vi "myRIO_BRig_FPGA_v3,2__PortC.vi"() -> ()   [LabVIEW 2014]
uses:
  <vilib>/rvi/FXPMathLib/FxpDiv/subVIs/nifxpmath_Div_SimConfig.ctl
  <vilib>/rvi/FXPMathLib/FxpSinAndCos/subVIs/nifxpmath_SinAndCos_SimConfig.ctl
  <vilib>/rvi/FXPMathLib/FxpDiv/simVIs/DllFxpDivTemp_sub.vi
  <vilib>/rvi/FXPMathLib/FxpSinAndCos/simVIs/DllFxpSinAndCosTemp_sub.vi
  <vilib>/rvi/Emulation/niFpgaGetClockAttributes.vi
  <vilib>/rvi/Emulation/niFpgaSctlEmulationGetInTimedLoop.vi
  <vilib>/rvi/Emulation/niFpgaEmulationReportErrorSimple.vi
  <vilib>/rvi/eio/common/nirviEmuTemplateMethod_errors.vi
  <vilib>/rvi/Emulation/niFpgaCriticalErrorInLSC.vi
  <vilib>/rvi/FXPMathLib/FxpDiv/XNode/nifxpmath_Div.xnode
  <vilib>/rvi/FXPMathLib/FxpMul/XNode/nifxpmath_Multiplier.xnode
  <vilib>/rvi/FXPMathLib/FxpSinAndCos/XNode/nifxpmath_SinAndCos.xnode
  <vilib>/rvi/FXPMathLib/FxpSub/XNode/nifxpmath_Sub.xnode
  <vilib>/eio/EIONode/EIONode.xnode
  <vilib>/rvi/FXPMathLib/sim/FxpSim.dll
panel:
  in  "AO0":i16
  in  "f_time_select":u32=173
  in  "laser_Nvalley":u32=100
  in  "laser_Npeak":u32=100
  in  "laserledMTrig":bool
  in  "tCycle_laser_wro":u32=100
  in  "tDelay_laser_wro":u32
  in  "tCycle_laser_rew":u32=100
  in  "tDelay_laser_rew":u32
  in  "laserResponse_reward_LED":bool
  in  "laserResponse_wrong_LED":bool
  out "SelectWrong":bool
  out "SelectReward":bool
  in  "laserResponse_wrong":bool
  in  "laserResponse_reward":bool
  in  "Left(F)_or_Right(T)":bool
  in  "ignoreWrong":bool
  in  "SelectionState":bool
  in  "laserMTrig":bool
  in  "FPGA_Stop":bool
  in  "audioTrigger_L":bool
  in  "audioTrigger_R":bool
  in  "audioFreq_L_Hz":u16=1000 min=1000 max=14000 step=1000
  in  "audioAmp_L":u16=1 min=1 max=32767 step=1
  in  "audioFreq_R_Hz":u16=1000 min=1000 max=14000 step=1000
  in  "audioAmp_R":u16=1 min=1 max=32767 step=1
  in  "A3_SL":bool
  in  "A1_SR":bool
  in  "Counts_Reset":bool
  out "A4_LickR":u32
  out "A2_LickL":u32
  in  "A6_Act":bool
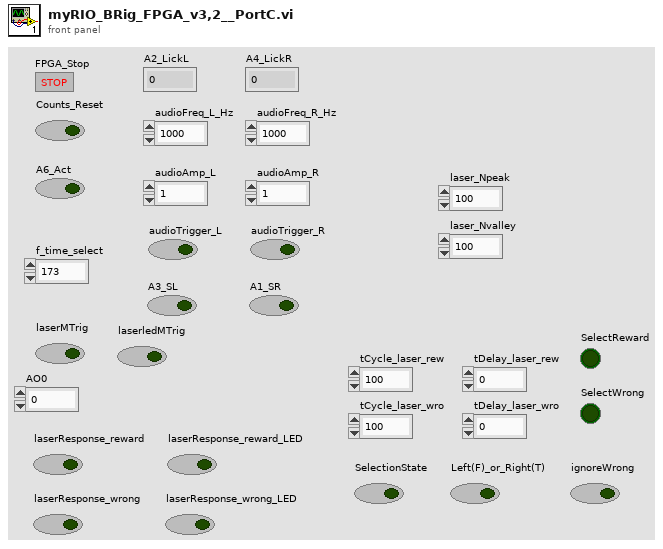
[diagram p1: front panel]
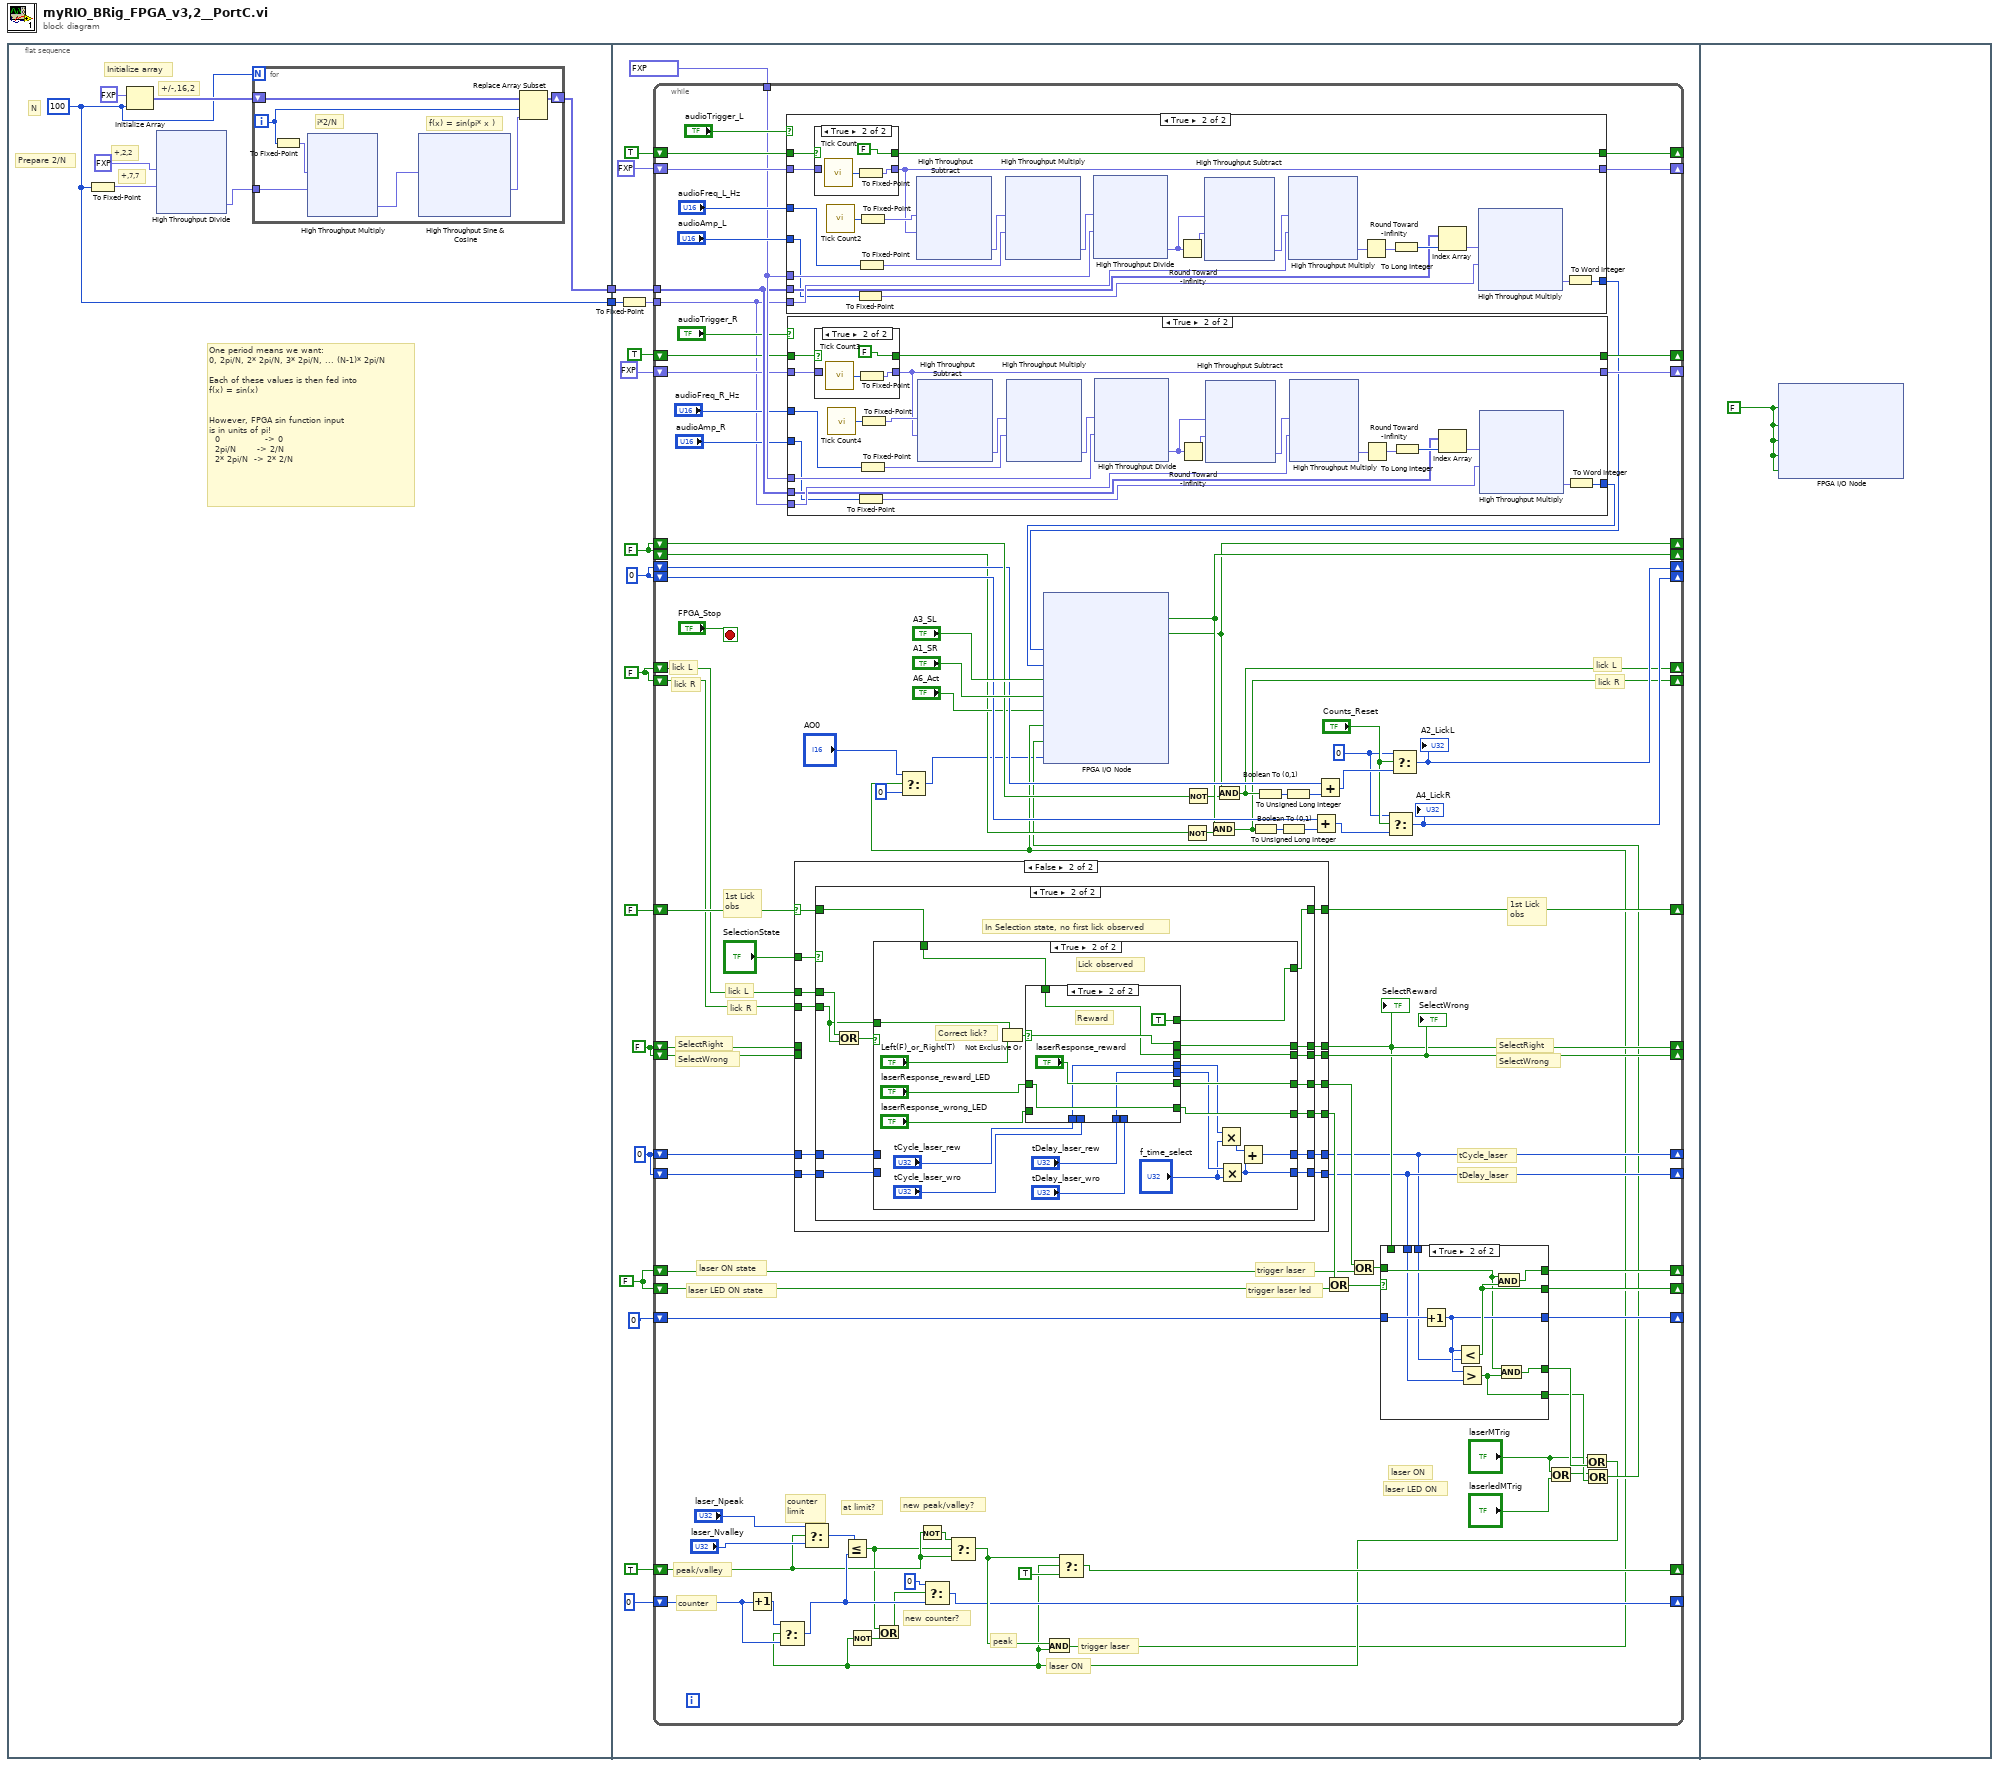
[diagram p0: block diagram]
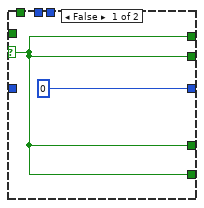
[diagram p2: hidden frame]
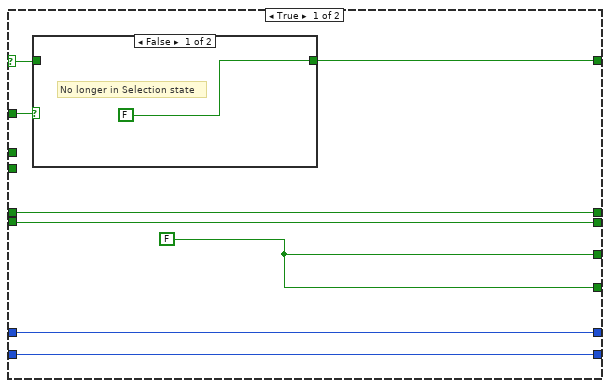
[diagram p3: hidden frame]
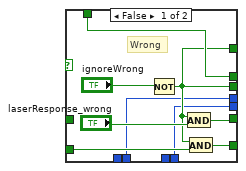
[diagram p7: hidden frame]
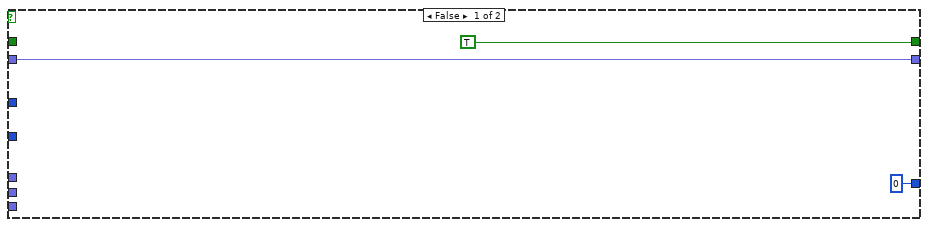
[diagram p8: hidden frame]
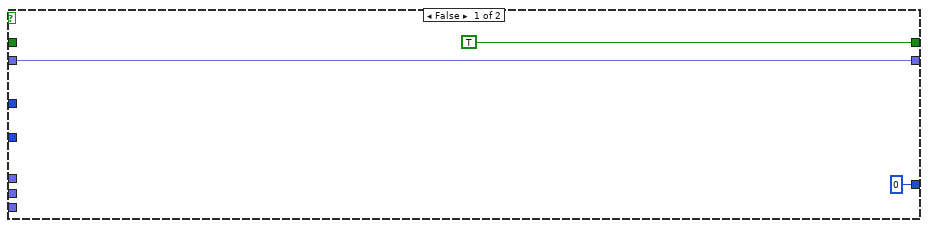
[diagram p10: hidden frame]
diagram:
  n1 = flat-sequence {
    tunnel: [w4] -> w2
    tunnel: [w3] -> w1
    tunnel: w2 -> [w86]
    tunnel: w1 -> [w88]
    frame #0 {
      w3 = 100 ("dimension size")
      # "N"
      # "+,7,7"
      # "+,2,2"
      # "+/-,16,2"
      # "Prepare 2/N"
      # "One period means we want:\n0, 2pi/N, 2* 2pi/N, 3* 2pi/N, ... (N-1)* 2pi/N\n\nEach of these values is then fed into\nf(x) = sin(x)\n\n\nHowever, FPGA sin function input\nis in units of pi!\n  0               -> 0\n  2pi/N       -> 2/N\n  2* 2pi/N  -> 2* 2/N"
      # "Initialize array"
      n2 = To Fixed-Point(number=w3) -> (fixed-point=w6:fxp<+,7,7>)  [unwired: 1 in]
      n3 = Initialize Array(fxp<+/-,16,2> 0.0 ("element"), w3) -> (w9:fxp<+/-,16,2>[])
      n4 = xnode "High Throughput Divide"("x"=fxp<+,2,2> 2.0, "y"=w6) -> ("x/y"=w5:fxp<+,27,0>)
      n5 = for {
        N: w3 -> [_]
        shift-right: [w42] -> w4
        shift-left: w9 -> [w43]
        tunnel: w5 -> [w38]
        i -> [w41]
        # "f(x) = sin(pi* x )"
        # "i*2/N"
        n6 = To Fixed-Point(number=w41) -> (fixed-point=w39:fxp<+,7,7>)  [unwired: 1 in]
        n7 = xnode ("High Throughput Multiply")("x"=w39, "y"=w38) -> ("x*y"=w37:fxp<+,34,7>)
        n8 = xnode "High Throughput Sine & Cosine"("x (pi)"=w37) -> ("sin(x)"=w40:fxp<+/-,16,2>)  [unwired: 1 out]
        n9 = Replace Array Subset(array=w43, new element=w40, index=w41) -> (w42:fxp<+/-,16,2>[])
      }
    }
    frame #1 {
      w76 = u32 0
      w78 = FALSE
      w77 = FALSE
      w81 = FALSE
      w82 = FALSE
      w83 = u32 0
      n10 = To Fixed-Point(number=w88) -> (fixed-point=w87:fxp<+,7,7>)  [unwired: 1 in]
      n11 = while {
        shift-right: [w178] -> _
        shift-left: TRUE -> [w182]
        shift-right: [w177] -> _
        shift-left: fxp<+,32,32> 0.0 -> [w181]
        tunnel: fxp<+,17,26> 40000000.0 -> [w176]
        tunnel: w87 -> [w169]
        tunnel: w86 -> [w175]
        shift-right: [w168] -> _
        shift-left: TRUE -> [w174]
        shift-right: [w167] -> _
        shift-left: fxp<+,32,32> 0.0 -> [w173]
        shift-right: [w144] -> _
        shift-left: w83 -> [w156]
        shift-right: [w147] -> _
        shift-left: w83 -> [w160]
        shift-right: [w148] -> _
        shift-left: w82 -> [w151]
        shift-right: [w145] -> _
        shift-left: w82 -> [w157]
        shift-right: [w142] -> _
        shift-left: FALSE -> [w141]
        shift-right: [w140] -> _
        shift-left: w81 -> [w138]
        shift-right: [w139] -> _
        shift-left: w81 -> [w137]
        shift-right: [w127] -> _
        shift-left: w77 -> [w129]
        shift-right: [w135] -> _
        shift-left: u32 0 -> [w136]
        shift-right: [w121] -> _
        shift-left: w78 -> [w133]
        shift-right: [w134] -> _
        shift-left: w78 -> [w132]
        shift-right: [w128] -> _
        shift-left: w77 -> [w125]
        shift-right: [w117] -> _
        shift-left: w76 -> [w120]
        shift-right: [w118] -> _
        shift-left: w76 -> [w119]
        shift-right: [w100] -> _
        shift-left: u32 0 -> [w111]
        shift-right: [w101] -> _
        shift-left: TRUE -> [w104]
        stop <- "FPGA_Stop" stop-if-true
        w153 = u32 0
        # "trigger laser"
        # "peak"
        # "laser ON"
        # "new peak/valley?"
        # "counter"
        # "peak/valley"
        # "new counter?"
        # "at limit?"
        # "counter\nlimit"
        # "tDelay_laser"
        # "tCycle_laser"
        # "laser LED ON"
        # "laser ON"
        # "laser LED ON state"
        # "laser ON state"
        # "SelectWrong"
        # "SelectRight"
        # "SelectWrong"
        # "SelectRight"
        # "lick R"
        # "lick L"
        # "1st Lick\nobs"
        # "1st Lick\nobs"
        # "lick R"
        # "lick L"
        # "lick R"
        # "lick L"
        # "trigger laser led"
        # "trigger laser"
        n12 = Increment(x=w111) -> (x+1=w109:u32)
        n13 = case shown="True" "audioTrigger_L" {
          tunnel: w182 -> [_ w360]
          tunnel: w181 -> [w336 w359]
          tunnel: "audioFreq_L_Hz" -> [_ w356]
          tunnel: w176 -> [_ w353]
          tunnel: [w336 w337] -> w177
          tunnel: [TRUE w350] -> w178
          tunnel: w169 -> [_ w349]
          tunnel: w175 -> [_ w344]
          tunnel: "audioAmp_L" -> [_ w342]
          tunnel: [i16 0 w339] -> w163
          frame False {
          }
          frame True {
            n14 = case shown="True" w360 {
              selector: w360 -> [w389 _]
              tunnel: [w389 FALSE] -> w350
              tunnel: w359 -> [w388 _]
              tunnel: [w388 w390] -> w337
              frame False {
              }
              frame True {
                n15 = call "Tick Count"() -> ("Tick Count(Ticks)"=w392:u32)
                n16 = To Fixed-Point(number=w392) -> (fixed-point=w390:fxp<+,32,32>)  [unwired: 1 in]
              }
            }
            n17 = call "Tick Count2"() -> ("Tick Count(Ticks)"=w358:u32)
            n18 = To Fixed-Point(number=w342) -> (fixed-point=w341:fxp<+,15,15>)  [unwired: 1 in]
            n19 = To Fixed-Point(number=w356) -> (fixed-point=w355:fxp<+,14,14>)  [unwired: 1 in]
            n20 = To Fixed-Point(number=w358) -> (fixed-point=w338:fxp<+,32,32>)  [unwired: 1 in]
            n21 = xnode "High Throughput Subtract"("x"=w338, "y"=w337) -> ("x-y"=w357:fxp<+,32,32>)
            n22 = xnode ("High Throughput Multiply")("x"=w357, "y"=w355) -> ("x*y"=w354:fxp<+,46,46>)
            n23 = xnode "High Throughput Divide"("x"=w354, "y"=w353) -> ("x/y"=w352:fxp<+,34,21>)
            n24 = Round Toward -Infinity(1:w352) -> (0:w351:fxp<+,21,21>)
            n25 = xnode "High Throughput Subtract"("x"=w352, "y"=w351) -> ("x-y"=w348:fxp<+,14,1>)
            n26 = xnode ("High Throughput Multiply")("x"=w348, "y"=w349) -> ("x*y"=w345:fxp<+,21,8>)
            n27 = Round Toward -Infinity(1:w345) -> (0:w347:fxp<+,8,8>)
            n28 = To Long Integer(number=w347) -> (32bit integer=w346:i32)
            n29 = Index Array(array=w344, index=w346) -> (element=w343:fxp<+/-,16,2>)
            n30 = xnode ("High Throughput Multiply")("x"=w343, "y"=w341) -> ("x*y"=w340:fxp<+/-,31,17>)
            n31 = To Word Integer(number=w340) -> (16bit integer=w339:i16)
          }
        }
        n32 = case shown="True" "audioTrigger_R" {
          tunnel: w174 -> [_ w301]
          tunnel: w173 -> [w277 w300]
          tunnel: "audioFreq_R_Hz" -> [_ w297]
          tunnel: w176 -> [_ w294]
          tunnel: [w277 w278] -> w167
          tunnel: [TRUE w291] -> w168
          tunnel: w169 -> [_ w290]
          tunnel: w175 -> [_ w285]
          tunnel: "audioAmp_R" -> [_ w283]
          tunnel: [i16 0 w280] -> w164
          frame False {
          }
          frame True {
            n33 = case shown="True" w301 {
              selector: w301 -> [w330 _]
              tunnel: [w330 FALSE] -> w291
              tunnel: w300 -> [w329 _]
              tunnel: [w329 w331] -> w278
              frame False {
              }
              frame True {
                n34 = call "Tick Count3"() -> ("Tick Count(Ticks)"=w333:u32)
                n35 = To Fixed-Point(number=w333) -> (fixed-point=w331:fxp<+,32,32>)  [unwired: 1 in]
              }
            }
            n36 = call "Tick Count4"() -> ("Tick Count(Ticks)"=w299:u32)
            n37 = To Fixed-Point(number=w283) -> (fixed-point=w282:fxp<+,15,15>)  [unwired: 1 in]
            n38 = To Fixed-Point(number=w297) -> (fixed-point=w296:fxp<+,14,14>)  [unwired: 1 in]
            n39 = To Fixed-Point(number=w299) -> (fixed-point=w279:fxp<+,32,32>)  [unwired: 1 in]
            n40 = xnode "High Throughput Subtract"("x"=w279, "y"=w278) -> ("x-y"=w298:fxp<+,32,32>)
            n41 = xnode ("High Throughput Multiply")("x"=w298, "y"=w296) -> ("x*y"=w295:fxp<+,46,46>)
            n42 = xnode "High Throughput Divide"("x"=w295, "y"=w294) -> ("x/y"=w293:fxp<+,34,21>)
            n43 = Round Toward -Infinity(1:w293) -> (0:w292:fxp<+,21,21>)
            n44 = xnode "High Throughput Subtract"("x"=w293, "y"=w292) -> ("x-y"=w289:fxp<+,14,1>)
            n45 = xnode ("High Throughput Multiply")("x"=w289, "y"=w290) -> ("x*y"=w286:fxp<+,21,8>)
            n46 = Round Toward -Infinity(1:w286) -> (0:w288:fxp<+,8,8>)
            n47 = To Long Integer(number=w288) -> (32bit integer=w287:i32)
            n48 = Index Array(array=w285, index=w287) -> (element=w284:fxp<+/-,16,2>)
            n49 = xnode ("High Throughput Multiply")("x"=w284, "y"=w282) -> ("x*y"=w281:fxp<+/-,31,17>)
            n50 = To Word Integer(number=w281) -> (16bit integer=w280:i16)
          }
        }
        n51 = case shown="False" w141 {
          selector: w141 -> [w201 w216]
          tunnel: "SelectionState" -> [w203 w218]
          tunnel: [w202 w217] -> w142
          tunnel: w138 -> [_ w215]
          tunnel: w137 -> [_ w214]
          tunnel: [w200 w213] -> w126
          tunnel: [w198 w212] -> w121
          tunnel: [w199 w211] -> w134
          tunnel: w133 -> [w198 _]
          tunnel: w132 -> [w199 _]
          tunnel: [w200 w210] -> w130
          tunnel: [w197 w209] -> w117
          tunnel: [w196 w208] -> w118
          tunnel: w120 -> [w197 w207]
          tunnel: w119 -> [w196 w206]
          frame True {
            w200 = FALSE
            n52 = case shown="False" w203 {
              tunnel: [FALSE w205] -> w202
              tunnel: w201 -> [_ w205]
              frame False {
                # "No longer in Selection state"
              }
              frame True {
                # "Already observed first lick, no other action"
              }
            }
          }
          frame False {
            n53 = case shown="True" w218 {
              tunnel: [w221 w231] -> w217
              tunnel: w216 -> [w221 w227]
              tunnel: w215 -> [_ w233]
              tunnel: w214 -> [_ w232]
              tunnel: [w221 w230] -> w213
              tunnel: [w221 w229] -> w212
              tunnel: [w221 w228] -> w211
              tunnel: [w221 w226] -> w210
              tunnel: [w220 w225] -> w209
              tunnel: [w219 w224] -> w208
              tunnel: w207 -> [w220 w223]
              tunnel: w206 -> [w219 w222]
              frame False {
                # "Not in Selection state"
              }
              frame True {
                # "In Selection state, no first lick observed"
                n54 = Or(x=w233, y=w232) -> (x .or. y?=w234:bool)
                n55 = case shown="True" w234 {
                  tunnel: w232 -> [_ w257]
                  tunnel: [w237 w250] -> w231
                  tunnel: [w237 w255] -> w230
                  tunnel: [w237 w254] -> w229
                  tunnel: [w237 w253] -> w228
                  tunnel: w227 -> [w237 w252]
                  tunnel: [w237 w251] -> w226
                  tunnel: [w236 w239] -> w225
                  tunnel: [w235 w238] -> w224
                  tunnel: w223 -> [w236 _]
                  tunnel: w222 -> [w235 _]
                  frame False {
                  }
                  frame True {
                    # "Correct lick?"
                    # "Lick observed"
                    n56 = Not Exclusive Or(1:"Left(F)_or_Right(T)", 2:w257) -> (0:w256:bool)
                    n57 = case shown="True" w256 {
                      selector: w256 -> [_ w273]
                      tunnel: [w264 "laserResponse_reward"] -> w255
                      tunnel: [w262 w269] -> w253
                      tunnel: [w266 w273] -> w254
                      tunnel: w252 -> [w266 w269]
                      tunnel: [w263 w271] -> w251
                      tunnel: [w262 TRUE] -> w250
                      tunnel: "laserResponse_reward_LED" -> [_ w271]
                      tunnel: "laserResponse_wrong_LED" -> [w261 _]
                      tunnel: "tCycle_laser_rew" -> [_ w268]
                      tunnel: "tCycle_laser_wro" -> [w259 _]
                      tunnel: "tDelay_laser_rew" -> [_ w270]
                      tunnel: "tDelay_laser_wro" -> [w260 _]
                      tunnel: [w260 w270] -> w242
                      tunnel: [w259 w268] -> w241
                      frame False {
                        # "Wrong"
                        n58 = Not(x="ignoreWrong") -> (.not. x?=w262:bool)
                        n59 = And(x=w262, y="laserResponse_wrong") -> (x .and. y?=w264:bool)
                        n60 = And(x=w262, y=w261) -> (x .and. y?=w263:bool)
                      }
                      frame True {
                        # "Reward"
                      }
                    }
                    n61 = Multiply(x=w241, y="f_time_select") -> (x*y=w243:u32)
                    n62 = Multiply(x=w242, y="f_time_select") -> (x*y=w238:u32)
                    n63 = Add(x=w243, y=w238) -> (x+y=w239:u32)
                  }
                }
              }
            }
          }
        }
        "SelectWrong" <- w134
        "SelectReward" <- w121
        n64 = Select(t="laser_Npeak", s=w104, f="laser_Nvalley") -> (s? t:f=w113:u32)
        n65 = Not(x=w104) -> (.not. x?=w105:bool)
        n66 = Not(x=w151) -> (.not. x?=w150:bool)
        n67 = Not(x=w157) -> (.not. x?=w146:bool)
        n68 = Or(x=w130, y=w129) -> (x .or. y?=w131:bool)
        n69 = Or(x=w126, y=w125) -> (x .or. y?=w124:bool)
        n70 = case shown="True" w131 {
          selector: w131 -> [w185 _]
          tunnel: w136 -> [_ w195]
          tunnel: [u32 0 w192] -> w135
          tunnel: [w185 w193] -> w127
          tunnel: [w185 w194] -> w128
          tunnel: w124 -> [_ w191]
          tunnel: [w185 w190] -> w122
          tunnel: [w185 w189] -> w123
          tunnel: w121 -> [_ _]
          tunnel: w118 -> [_ w188]
          tunnel: w117 -> [_ w187]
          frame False {
          }
          frame True {
            n71 = Increment(x=w195) -> (x+1=w192:u32)
            n72 = Less?(x=w192, y=w187) -> (x < y?=w193:bool)
            n73 = Greater?(x=w192, y=w188) -> (0:w190:bool)
            n74 = And(x=w191, y=w193) -> (x .and. y?=w194:bool)
            n75 = And(x=w191, y=w190) -> (x .and. y?=w189:bool)
          }
        }
        n76 = Or(x="laserMTrig", y="laserledMTrig") -> (x .or. y?=w115:bool)
        n77 = Or(x="laserMTrig", y=w123) -> (x .or. y?=w98:bool)
        n78 = Select(t=w109, s=w98, f=w111) -> (s? t:f=w108:u32)
        n79 = Less Or Equal?(x=w113, y=w108) -> (x <= y?=w97:bool)
        n80 = Not(x=w98) -> (.not. x?=w99:bool)
        n81 = Or(x=w97, y=w99) -> (x .or. y?=w96:bool)
        n82 = Select(t=u32 0, s=w96, f=w108) -> (s? t:f=w100:u32)
        n83 = Select(t=w105, s=w97, f=w104) -> (s? t:f=w103:bool)
        n84 = And(x=w103, y=w98) -> (x .and. y?=w95:bool)
        n85 = Select(t="AO0", s=w95, f=i16 0) -> (s? t:f=w93:i16)
        n86 = Select(t=w103, s=w98, f=TRUE) -> (s? t:f=w101:bool)
        n87 = Or(x=w115, y=w122) -> (x .or. y?=w110:bool)
        n88 = xnode "FPGA I/O Node"("AudioOut/Left"=w163, "AudioOut/Right"=w164, "ConnectorC/DIO3"="A3_SL", "ConnectorC/DIO1"="A1_SR", "ConnectorC/DIO6"="A6_Act", "ConnectorC/DIO0"=w95, "ConnectorC/DIO7"=w110, "ConnectorC/AO0"=w93) -> ("ConnectorC/DIO4"=w148:bool, "ConnectorC/DIO2"=w145:bool)  [unwired: 10 in, 10 out]
        n89 = And(x=w148, y=w150) -> (x .and. y?=w139:bool)
        n90 = And(x=w145, y=w146) -> (x .and. y?=w140:bool)
        n91 = Boolean To (0,1)(Boolean=w139) -> (0, 1=w162:i16)
        n92 = Boolean To (0,1)(Boolean=w140) -> (0, 1=w159:i16)
        n93 = To Unsigned Long Integer(number=w162) -> (unsigned 32bit integer=w161:u32)
        n94 = To Unsigned Long Integer(number=w159) -> (unsigned 32bit integer=w158:u32)
        n95 = Add(x=w160, y=w161) -> (x+y=w149:u32)
        n96 = Add(x=w156, y=w158) -> (x+y=w155:u32)
        n97 = Select(t=w153, s="Counts_Reset", f=w149) -> (s? t:f=w147:u32)
        "A4_LickR" <- w147
        n98 = Select(t=w153, s="Counts_Reset", f=w155) -> (s? t:f=w144:u32)
        "A2_LickL" <- w144
      }
    }
    frame #2 {
      w393 = FALSE ("ConnectorA/DIO3")
      n99 = xnode "FPGA I/O Node"("ConnectorC/DIO3"=w393, "ConnectorC/DIO1"=w393, "ConnectorC/DIO0"=w393, "ConnectorC/DIO6"=w393, "ConnectorC/DIO7"=w393) -> ()  [unwired: 5 in, 5 out]
    }
  }
